vi "Stop Core.vi"(10 "final error code":i32, 11 "MSS Target Actor in":refnum<class "MSS Target Actor.lvclass">) -> (3 "MSS Target Actor out":refnum<class "MSS Target Actor.lvclass">)   [LabVIEW 2024, in "MSS Target Actor.lvlib" / "MSS Target Actor.lvclass"]
doc: "(<B>Filename</B>: Actor Framework.lvlib:Actor.lvclass:Stop Core.vi)\n\nDefines what the actor does before it stops. Use the <B>final error code</B> input to determine whether the actor shut down in response to an error.\n\nBy default, this method passes the Stop message along to all auto-stop nested actors. A descendant class may override this method to define additional behavior, such as shutting down any processes the actor initiated in its override of the Actor Core method."
uses:
  MSS Target Actor.lvclass
  MSS Target Actor.lvclass/MSS Target Actor.ctl
  <vilib>/ActorFramework/Actor/Actor.lvclass
  MSS/MSS.lvclass
  Reply-Msg-DataSocket/Reply Msg DataSocket/Reply Msg DataSocket.lvclass
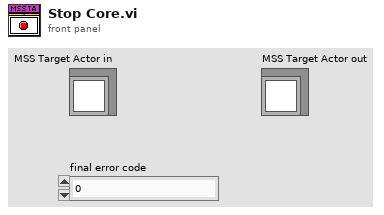
[diagram p1: front panel]
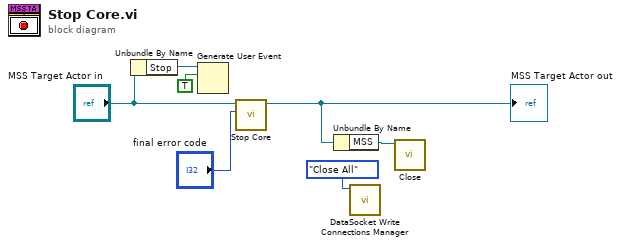
[diagram p0: block diagram]
diagram:
  n1 = Unbundle By Name("MSS Target Actor in") -> ("Stop"=w3:refnum<user-event>)
  n2 = Generate User Event(user event=w3, event data cluster=TRUE ("event data")) -> ()  [unwired: 2 in, 2 out]
  n3 = call-parent "Stop Core.vi"("final error code"="final error code", "Actor in"="MSS Target Actor in") -> ("Actor out"=w6:refnum<class "MSS Target Actor.lvclass">)  [unwired: 9 in]
  "MSS Target Actor out" <- w6
  n4 = Unbundle By Name(w6) -> ("MSS"=w5:refnum<class "MSS.lvclass">)
  n5 = call "DataSocket Write Connections Manager.vi"("Action"=enum16{"Get", "Close", "Close All"}."Close All") -> ()  [unwired: 9 in, 2 out]
  n6 = call "Close.vi"("MSS in"=w5) -> ()  [unwired: 9 in, 2 out]
